vi "NI_USB-6501_semafor.vi"() -> ()   [LabVIEW 2013]
panel:
  out "P2":u8[](array[numeric]) format="%x"
  out "P1":u8[](array[numeric]) format="%x"
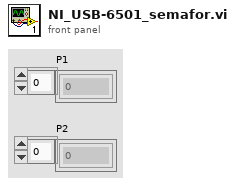
[diagram p1: front panel]
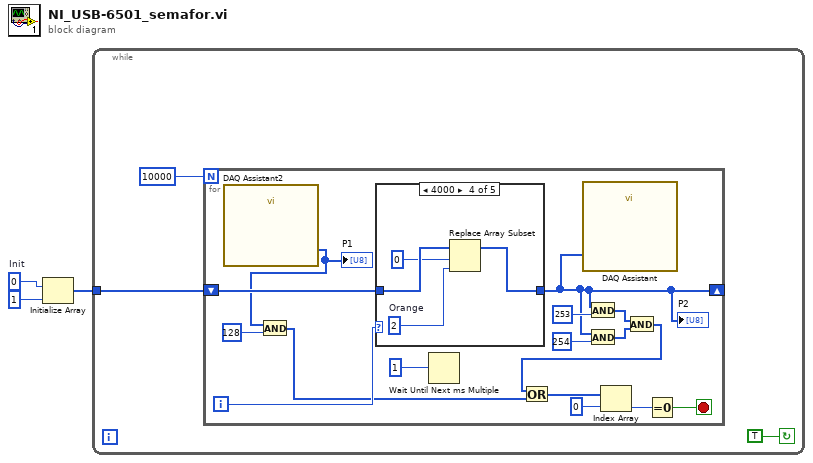
[diagram p0: block diagram]
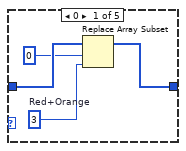
[diagram p2: hidden frame]
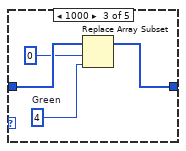
[diagram p4: hidden frame]
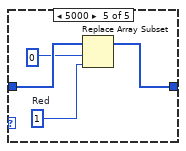
[diagram p5: hidden frame]
diagram:
  w3 = u8 0  # Init
  n1 = Initialize Array(w3, u8 1) -> (w2:u8[])
  n2 = while {
    tunnel: w2 -> [w5]
    stop <- TRUE continue-if-true
    n3 = for {
      N: u32 10000 -> [_]
      shift-right: [w14] -> _
      shift-left: w5 -> [w22]
      i -> [w20]
      stop <- w13 stop-if-true
      n4 = call "DAQ Assistant2"() -> ("data"=w15:u32[])  [unwired: 17 in, 2 out]
      "P1" <- w15
      n5 = And(x=w15, y=u8 128) -> (x .and. y?=w9:u32[])
      n6 = case shown="4000" w20 {
        tunnel: w22 -> [w26 w27 w31 w35 w39]
        tunnel: [w25 w27 w30 w34 w37] -> w14
        frame 0 {
          w24 = u8 3  # Red+Orange
          n7 = Replace Array Subset(array=w26, new element=w24, index=u8 0) -> (w25:u8[])
        }
        frame 1, Default {
        }
        frame 1000 {
          w29 = u8 4  # Green
          n8 = Replace Array Subset(array=w31, new element=w29, index=u8 0) -> (w30:u8[])
        }
        frame 4000 {
          w33 = u8 2  # Orange
          n9 = Replace Array Subset(array=w35, new element=w33, index=u8 0) -> (w34:u8[])
        }
        frame 5000 {
          w38 = u8 1  # Red
          n10 = Replace Array Subset(array=w39, new element=w38, index=u8 0) -> (w37:u8[])
        }
      }
      "P2" <- w14
      n11 = Wait Until Next ms Multiple(millisecond multiple=1) -> ()  [unwired: 1 out]
      n12 = call "DAQ Assistant"("data"=w14) -> ()  [unwired: 17 in, 2 out]
      n13 = And(x=w14, y=u8 253) -> (x .and. y?=w12:u8[])
      n14 = And(x=w14, y=u8 254) -> (x .and. y?=w11:u8[])
      n15 = And(x=w12, y=w11) -> (x .and. y?=w8:u8[])
      n16 = Or(x=w8, y=w9) -> (x .or. y?=w10:u32[])
      n17 = Index Array(array=w10, index=0) -> (element=w7:u32)
      n18 = Equal To 0?(x=w7) -> (x = 0?=w13:bool)
    }
  }
